vi "libssh2_knownhost_checkp - unknown host - returns not found.vi"() -> ()   [LabVIEW 2017, in "unit_tests.lvlib"]
uses:
  unit_tests.lvlib
  libssh2/Host Key Check Result.ctl
  libssh2/libssh2_init_default.vi
  libssh2/libssh2_session_init_ex.vi
  libssh2/libssh2.lvlib
  <vilib>/PNR/Transparent Assertions/Transparent Assertions/Transparent Assertions.lvlib
panel:
  out "error out":errorcluster
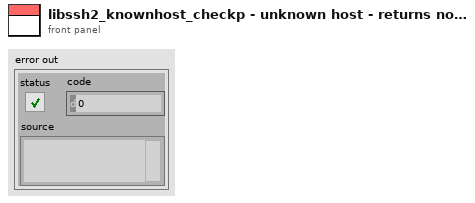
[diagram p1: front panel]
types:
  T1 = typedef "libssh2.lvlib/Host Key Check Result.ctl" = enum16{"Match", "Mismatch", "Not Found", "Failure"}
  T2 = typedef "libssh2.lvlib/Session Refnum.ctl" = refnum<k1>
  T3 = typedef "libssh2.lvlib/Host Key Database Refnum.ctl" = refnum<k1>
  T4 = typedef "libssh2.lvlib/Host Key Refnum.ctl" = refnum<k1>
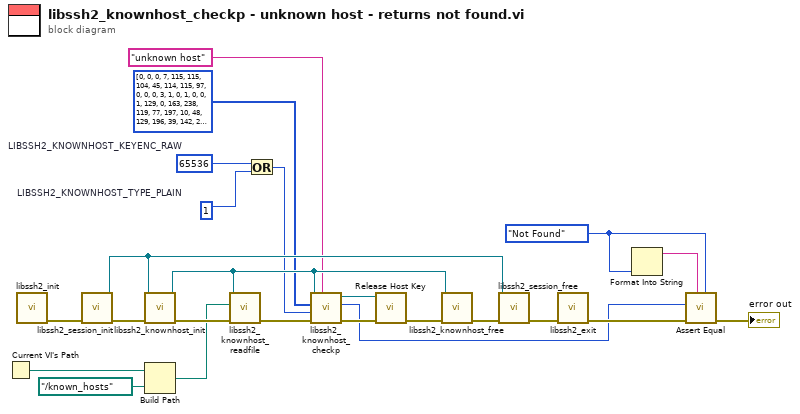
[diagram p0: block diagram]
diagram:
  w4 = Host_Key_Check_Result."Not Found" ("result")
  w9 = 1  # LIBSSH2_KNOWNHOST_TYPE_PLAIN
  w10 = 65536  # LIBSSH2_KNOWNHOST_KEYENC_RAW
  n1 = Current VI's Path() -> (path=w15:path)
  n2 = call-poly "libssh2_init.vi"() -> ("error out"=w23:errorcluster)  [unwired: 11 in]
  n3 = call "libssh2_session_init.vi"("error in (no error)"=w23) -> ("error out"=w22:errorcluster, "session"=w19:T2)  [unwired: 9 in]
  n4 = call "libssh2_knownhost_init.vi"("error in (no error)"=w22, "session"=w19) -> ("error out"=w17:errorcluster, "host key database"=w11:T3)  [unwired: 8 in]
  n5 = Build Path(base path=w15, name or relative path=path "../known_hosts" ("filename")) -> (appended path=w13:path)
  n6 = call "libssh2_knownhost_readfile.vi"("error in (no error)"=w17, "filename"=w13, "host key database"=w11) -> ("error out"=w16:errorcluster)  [unwired: 7 in, 1 out]
  n7 = Or(x=w10, y=w9) -> (x .or. y?=w8:i32)
  n8 = call "libssh2_knownhost_checkp.vi"("host"="unknown host", "error in (no error)"=w16, "typemask"=w8, "key"=u8[] [0, 0, 0, 7, 115, 115, 104, 45, 114, 115, 97, 0, 0, 0, 3, 1, 0, 1, 0, 0, 1, 129, 0, 163, 238, 119, 77, 197, 10, 48, 129, 196, 39, 142, 200, 92, 46, 186, 143, 18, 40, 169, 134, 123, 126, 85, 52, 239, 12, 254, 166, 28, 18, 253, 143, 86, 141, 82, 70, 56, 81, 237, 96, 191, 9, 198, 45, 89, 78, 132, 103, 152, 174, 118, 90, 50, 4, 74, 235, 227, 202, 9, 69, 218, 13, 176, 187, 170, 214, 214, 242, 2, 36, 132, 190, 218, 24, 43, 14, 175, 240, 185, 233, 34, 76, 203, 240, 66, 101, 252, 93, 214, 117, 179, 0, 236, 82, 12, 248, 21, 178, 103, 171, 56, 22, 31, 54, 169, 109, 87, 223, 225, 88, 42, 129, 203, 2, 13, 33, 31, 185, 116, 136, 58, 37, 50, 123, 218, 151, 4, 164, 72, 220, 98, 5, 228, 19, 102, 4, 21, 117, 117, 36, 121, 236, 42, 6, 203, 88, 217, 97, 73, 202, 155, 217, 73, 178, 70, 68, 50, 202, 212, 75, 180, 191, 183, 241, 49, 177, 147, 16, 159, 150, 99, 190, 229, 159, 2, 73, 35, 88, 236, 104, 157, 140, 194, 25, 237, 14, 51, 50, 48, 54, 159, 89, 198, 174, 84, 195, 147, 60, 3, 10, 204, 62, 194, 161, 79, 25, 0, 53, 239, 215, 39, 124, 101, 142, 89, 21, 107, 186, 61, 122, 207, 165, 242, 191, 27, 227, 39, 6, 243, 211, 4, 25, 239, 149, 202, 230, 210, 146, 111, 177, 77, 201, 226, 4, 179, 132, 211, 226, 57, 62, 75, 135, 97, 61, 224, 20, 11, 156, 190, 108, 54, 34, 173, 136, 12, 224, 96, 187, 184, 73, 243, 182, 118, 114, 105, 85, 144, 236, 29, 252, 212, 2, 184, 65, 218, 240, 183, 157, 89, 168, 76, 74, 109, 10, 83, 80, 217, 254, 18, 58, 168, 79, 11, 234, 54, 62, 36, 171, 30, 80, 80, 34, 52, 78, 20, 191, 98, 67, 177, 36, 37, 230, 61, 69, 153, 110, 24, 233, 10, 14, 122, 139, 237, 154, 7, 160, 166, 43, 98, 70, 134, 126, 123, 43, 153, 163, 208, 195, 93, 5, 112, 56, 253, 105, 240, 31, 165, 232, 61, 98, 115, 43, 147, 114, 187, 108, 193, 222, 112, 25, 167, 228, 185, 134, 148, 44, 250, 157, 111, 55, 95, 240, 178, 57] ("unsigned byte array"), "host key database"=w11) -> ("error out"=w12:errorcluster, "result"=w5:T1, "host key"=w6:T4)  [unwired: 4 in]
  n9 = call "Release Host Key.vi"("error in (no error)"=w12, "host key"=w6) -> ("error out"=w7:errorcluster)  [unwired: 9 in]
  n10 = call "libssh2_knownhost_free.vi"("error in (no error)"=w7, "host key database"=w11) -> ("error out"=w18:errorcluster)  [unwired: 9 in]
  n11 = call "libssh2_session_free.vi"("error in (no error)"=w18, "session"=w19) -> ("error out"=w21:errorcluster)  [unwired: 9 in]
  n12 = call "libssh2_exit.vi"("error in (no error)"=w21) -> ("error out"=w20:errorcluster)  [unwired: 10 in]
  n13 = Format Into String(w4) -> (resulting string=w3:string)  [unwired: 3 in, 1 out]
  n14 = call <vilib>:"Assert Equal.vi"("Expected"=w4, "Message (\"\")"=w3, "error in (no error)"=w20, "Actual"=w5) -> ("error out"=→"error out":errorcluster)  [unwired: 7 in]
